vi "BB_CameraIssue HTTP Request from MJPG-Streamer.vi"(8 "error in (no error)":errorcluster, 9 "remote port or service name":u16=5800, 10 "Request":string, 11 "address":string) -> (0 "error out":errorcluster, 2 "Authenticated request":string, 3 "connection ID (dup)":refnum<k5>)   [LabVIEW 2016]
doc: "This VI issues the given http request with the required added information and authentication. It cycles through an array of predetermined username, password combinations that we expect the users to have at any point in time. If none of the username, password combinations work, this VI returns an \"Unknown user or password\" error.\n\nThis software is licensed. Open the labview\\readme\\WPI Robotics Library Open Source License.txt file for more information."
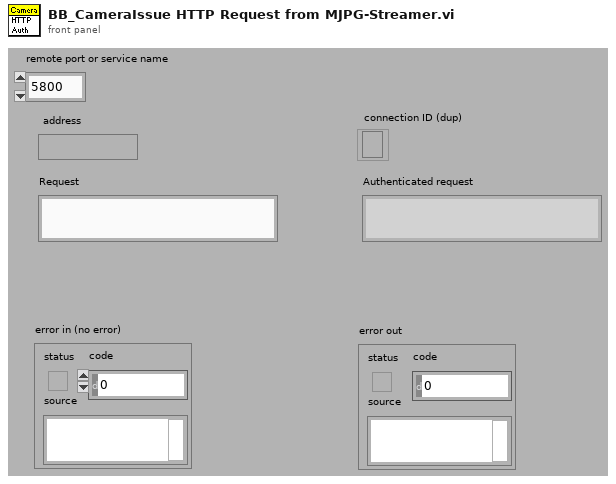
[diagram p1: front panel]
types:
  T1 = enum16{"Standard", "Buffered", "CRLF", "Immediate"}
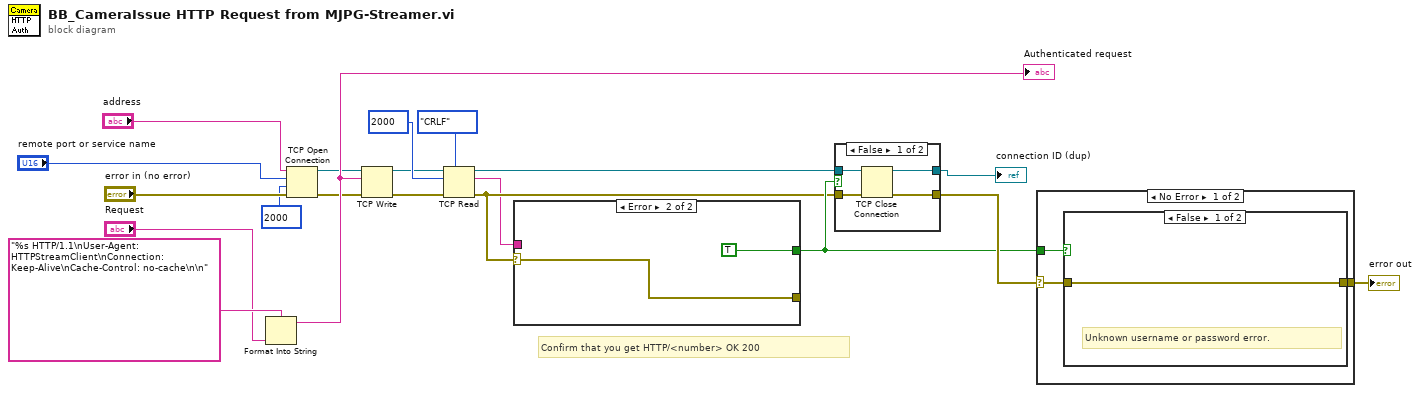
[diagram p0: block diagram]
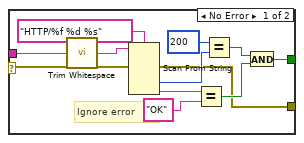
[diagram p3: hidden frame]
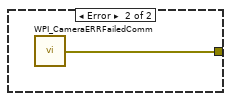
[diagram p5: hidden frame]
diagram:
  # "Confirm that you get HTTP/<number> OK 200"
  n1 = Format Into String(format string="%s HTTP/1.1\nUser-Agent: HTTPStreamClient\nConnection: Keep-Alive\nCache-Control: no-cache\n\n", "Request") -> (resulting string=w14:string)  [unwired: 2 in, 1 out]
  "Authenticated request" <- w14
  n2 = TCP Open Connection(address="address", remote port or service name="remote port or service name", timeout ms (60000)=2000, error in (no error)="error in (no error)") -> (connection ID=w6:refnum<k5>, error out=w5:errorcluster)  [unwired: 1 out]
  n3 = TCP Write(connection ID=w6, data in=w14, error in (no error)=w5) -> (connection ID out=w8:refnum<k5>, error out=w7:errorcluster)  [unwired: 2 out]
  n4 = TCP Read(connection ID=w8, bytes to read=2000, error in (no error)=w7, 7:T1."CRLF" ("mode (standard)")) -> (connection ID out=w4:refnum<k5>, data out=w1:string, error out=w3:errorcluster)  [unwired: 1 out]
  n5 = case shown="Error" w3 {
    selector: w3 -> [w24 w34]
    tunnel: [w25 TRUE] -> w16
    tunnel: [w23 w34] -> _
    tunnel: w1 -> [w21 _]
    frame No Error {
      # "Ignore error"
      n6 = call <vilib>:"Trim Whitespace.vi"("string"=w21) -> ("trimmed string"=w22:string)  [unwired: 1 in]
      n7 = Scan From String(format string="HTTP/%f %d %s", input string=w22, error in=w24) -> (error out=w23:errorcluster, output 2=w31:i32, output 3=w29:string)  [unwired: 1 in, 6 out]
      n8 = Equal?(x=w29, y="OK" ("format string")) -> (x = y?=w27:bool)
      n9 = Equal?(x=200, y=w31) -> (x = y?=w26:bool)
      n10 = And(x=w26, y=w27) -> (x .and. y?=w25:bool)
    }
    frame Error {
    }
  }
  n11 = case shown="False" w16 {
    tunnel: w4 -> [w38 w40]
    tunnel: w3 -> [w37 w39]
    tunnel: [w36 w40] -> w13
    tunnel: [w35 w39] -> w17
    frame False {
      n12 = TCP Close Connection(connection ID=w38, error in (no error)=w37) -> (connection ID out=w36:refnum<k5>, error out=w35:errorcluster)  [unwired: 1 out]
    }
    frame True {
    }
  }
  "connection ID (dup)" <- w13
  n13 = case shown="No Error" w17 {
    selector: w17 -> [w41 _]
    tunnel: w16 -> [w43 _]
    tunnel: [w42 w46] -> w15
    frame No Error {
      n14 = case shown="False" w43 {
        tunnel: [w44 w45] -> w42
        tunnel: w41 -> [w44 w45]
        frame False {
          # "Unknown username or password error."
        }
        frame True {
        }
      }
    }
    frame Error {
      n15 = call <vilib>:"WPI_CameraERRFailedComm.vi"() -> ("error out"=w46:errorcluster)
    }
  }
  "error out" <- w15
